vi "gjson_Flatten.vi"(5 "Encap'd by Array?":bool=TRUE, 7 "FlattenedData":string, 8 "error in":errorcluster, 9 "offset (0)":i32, 10 "Variant":variant, 11 "JSON String In":string) -> (0 "error out":errorcluster, 1 "offset out":i32, 3 "JSON String Out":string)   [LabVIEW 2015, in "Json2Labv.lvlib"]
doc: "This recursive VI is the core engine responsible for converting the LabVIEW cluster into an JSON string. \n\nThe VI identifies the top level datatype of the input variant and recursively calls itself when an encapsulaing datatype is found (ie cluster or array). When a fundamental item is found (integer, boolean, etc) it is converted to text and given tags with appropriate attributes and hierarchy."
uses:
  Json2Labv.lvlib
  <vilib>/Utility/VariantDataType/VariantType.lvlib
  <vilib>/Utility/Data Type/NI_Data Type.lvlib
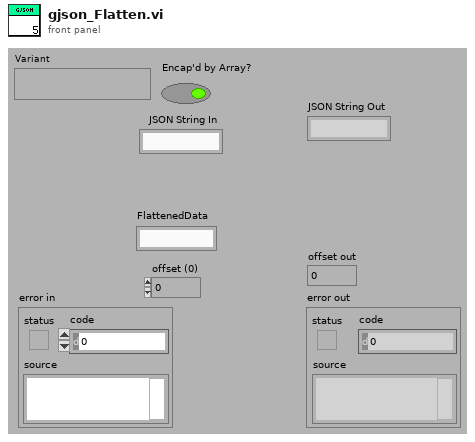
[diagram p1: front panel]
types:
  T1 = typedef "NI_Data Type.lvlib/Data Type.ctl" = enum8{"Invalid Type", "Void", "I8", "I16", "I32", "I64", "U8", "U16", "U32", "U64", "Single Float", "Double Float", "Extended Float", "Single Complex", "Double Complex", "Extended Complex", "Enum U8", "Enum U16", "Enum U32", "Enum U64", "Single Float With Unit", "Double Float With Unit", "Extended Float With Unit", "Single Complex with Unit", "Double Complex with Unit", "Extended Complex with Unit", "Boolean", "String", "Path", "Picture", "Tag", "Array", "Cluster", "Variant", "LV Variant", "Waveform", "Timestamp", "Digital Waveform", "Digital Data", "ExpressData", "Refnum", "External Data", "VI", "Poly VI", "LabVIEW Class Instance", "Fixed Point"}
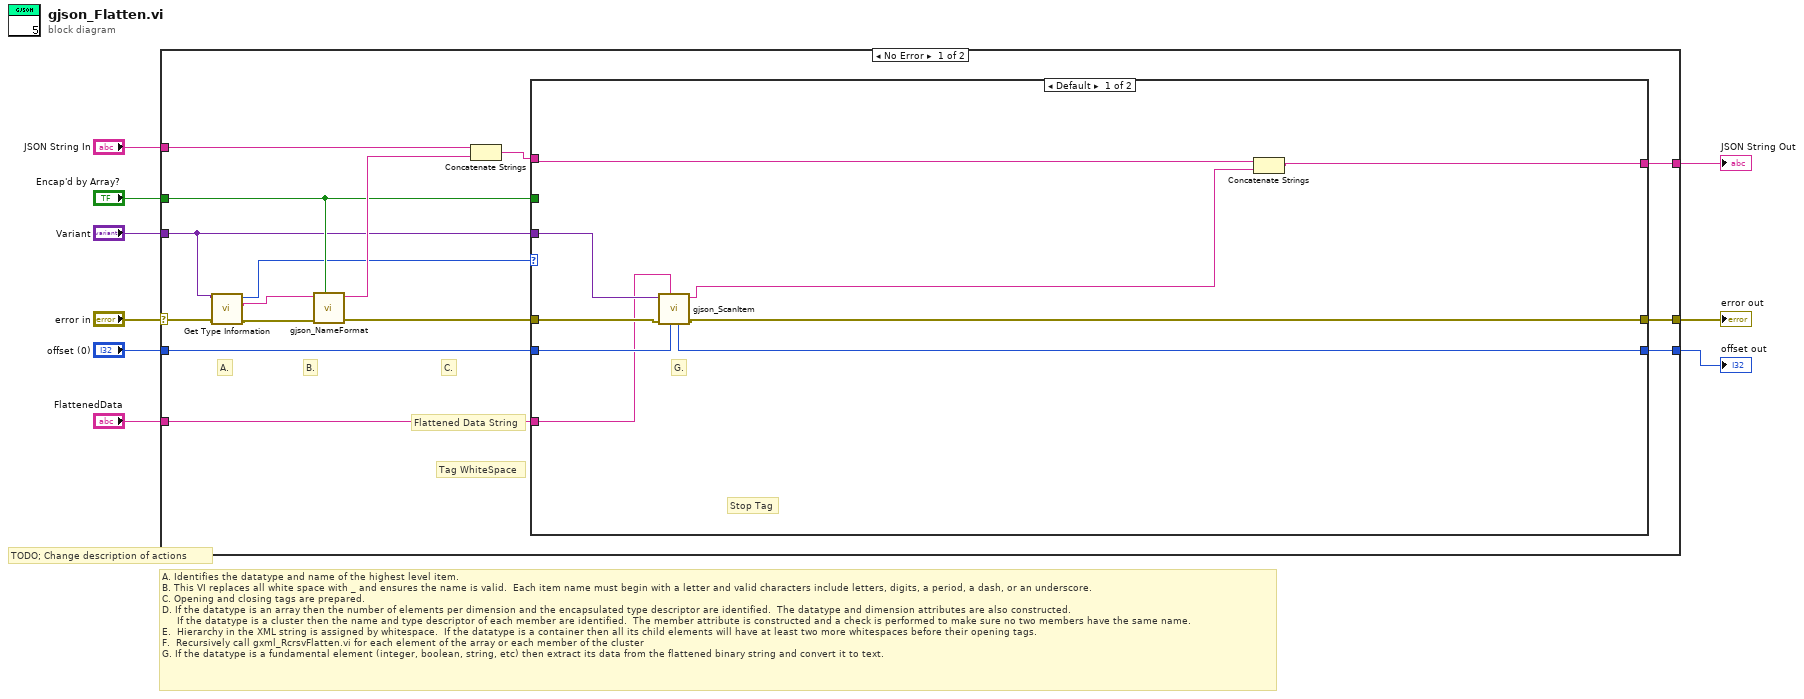
[diagram p0: block diagram]
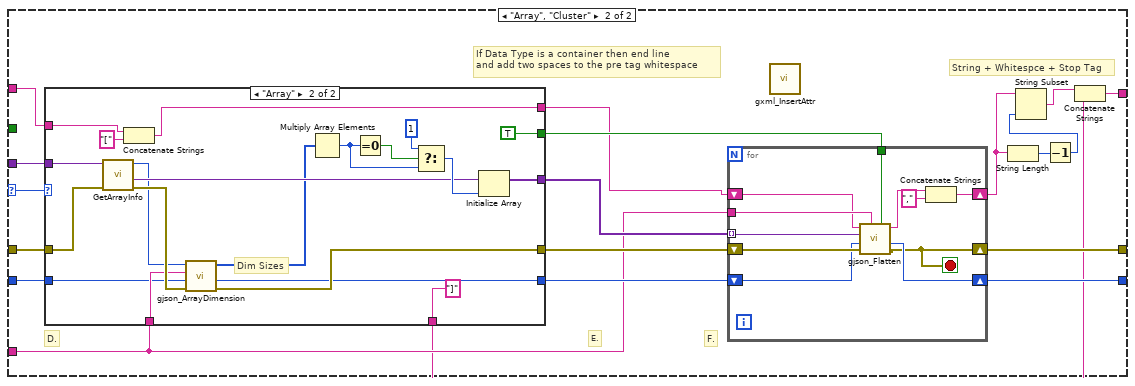
[diagram p2: hidden frame]
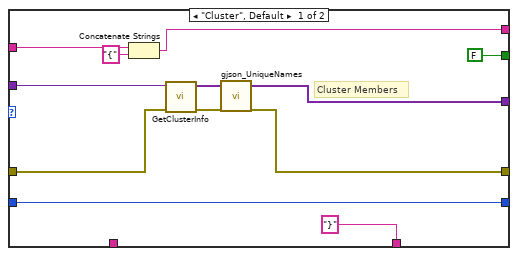
[diagram p3: hidden frame]
diagram:
  # "TODO; Change description of actions"
  # "A. Identifies the datatype and name of the highest level item.\nB. This VI replaces all white space with _ and ensures the name is valid.  Each item name must begin with a letter and valid characters include letters, digits, a period, a dash, or an underscore.\nC. Opening and closing tags are prepared.\nD. If the datatype is an array then the number of elements per dimension and the encapsulated type descriptor are identified.  The datatype and dimension attributes are also constructed.\n     If the datatype is a cluster then the name and type descriptor of each member are identified.  The member attribute is constructed and a check is performed to make sure no two members have the same name.\nE.  Hierarchy in the XML string is assigned by whitespace.  If the datatype is a container then all its child elements will have at least two more whitespaces before their opening tags.\nF.  Recursively call gxml_RcrsvFlatten.vi for each element of the array or each member of the cluster\nG. If the datatype is a fundamental element (integer, boolean, string, etc) then extract its data from the flattened binary string and convert it to text."
  n1 = case shown="No Error" "error in" {
    selector: "error in" -> [w13 w98]
    tunnel: [w24 w98] -> w9
    tunnel: [w22 w97] -> w6
    tunnel: [w23 w96] -> w3
    tunnel: "JSON String In" -> [w17 w97]
    tunnel: "Encap'd by Array?" -> [w15 _]
    tunnel: "offset (0)" -> [w20 w96]
    tunnel: "Variant" -> [w14 _]
    tunnel: "FlattenedData" -> [w19 _]
    frame No Error {
      # "C."
      # "B."
      # "A."
      # "Flattened Data String"
      # "Tag WhiteSpace"
      n2 = call <vilib>:"Get Type Information.vi"("error in (no error)"=w13, "Variant"=w14) -> ("error out"=w10:errorcluster, "Name"=w11:string, "Type"=w12:T1)  [unwired: 5 in, 2 out]
      n3 = call "gjson_NameFormat.vi"("Encap'd by Array?"=w15, "error in"=w10, "JSON String"=w11) -> ("error out"=w18:errorcluster, "JSON_String"=w16:string)  [unwired: 7 in]
      n4 = Concatenate Strings(w17, w16) -> (w21:string)
      n5 = case shown="Default" w12 {
        selector: w12 -> [_ w47]
        tunnel: w14 -> [w29 w52]
        tunnel: w18 -> [w32 w51]
        tunnel: [w27 w40] -> w22
        tunnel: w20 -> [w31 w50]
        tunnel: [w33 w46] -> w24
        tunnel: [w30 w45] -> w23
        tunnel: w21 -> [w25 w42]
        tunnel: w15 -> [_ _]
        tunnel: w19 -> [w28 w39]
        frame Default {
          # "G."
          # "Stop Tag"
          n6 = call "gjson_ScanItem.vi"("Offset In"=w31, "FlattenedData"=w28, "error in"=w32, "variant"=w29) -> ("error out"=w33:errorcluster, "DataString"=w26:string, "Offset Out"=w30:i32)  [unwired: 4 in, 1 out]
          n7 = Concatenate Strings(w25, w26) -> (w27:string)
        }
        frame "Array", "Cluster" {
          # "E."
          # "F."
          # "D."
          # "If Data Type is a container then end line\nand add two spaces to the pre tag whitespace"
          # "String + Whitespce + Stop Tag"
          n8 = case shown="\"Array\"" w47 {
            tunnel: w52 -> [w61 w77]
            tunnel: w51 -> [w62 w78]
            tunnel: w50 -> [w63 w65]
            tunnel: [w58 w84] -> w49
            tunnel: [w57 w71] -> w48
            tunnel: [FALSE TRUE] -> w44
            tunnel: [w63 w70] -> w43
            tunnel: w39 -> [_ w66]
            tunnel: w42 -> [w56 w74]
            tunnel: [w54 w73] -> w41
            tunnel: ["}" ("string") "]" ("string")] -> w34
            frame "Cluster", Default {
              # "Cluster Members"
              n9 = Concatenate Strings(w56, "{" ("string")) -> (w54:string)
              n10 = call <vilib>:"GetClusterInfo.vi"("error in (no error)"=w62, "Variant"=w61) -> ("error out"=w59:errorcluster, "Cluster Elements"=w60:variant[])  [unwired: 8 in]
              n11 = call "gjson_UniqueNames.vi"("error in"=w59, "Cluster Elements"=w60) -> ("error out"=w57:errorcluster, "Cluster Elements Out"=w58:variant[])  [unwired: 8 in]
            }
            frame "Array" {
              # "Dim Sizes"
              n12 = call <vilib>:"GetArrayInfo.vi"("error in (no error)"=w78, "Variant"=w77) -> ("error out"=w68:errorcluster, "ArrayElement"=w76:variant, "NDims"=w67:i32)  [unwired: 6 in, 1 out]
              n13 = Concatenate Strings(w74, "[" ("string")) -> (w73:string)
              n14 = call "gjson_ArrayDimension.vi"("error in"=w68, "offset (0)"=w65, "Flattened Data String"=w66, "Dimensions"=w67) -> ("error out"=w71:errorcluster, "offset"=w70:i32, "ArrayDimensions"=w69:i32[])  [unwired: 4 in, 1 out]
              n15 = Multiply Array Elements(1:w69) -> (0:w82:i32)
              n16 = Equal To 0?(x=w82) -> (x = 0?=w83:bool)
              n17 = Select(t=1, s=w83, f=w82) -> (s? t:f=w80:i32)
              n18 = Initialize Array(w76, w80) -> (w84:variant[])
            }
          }
          n19 = for {
            shift-right: [w86] -> w38
            shift-left: w41 -> [w89]
            shift-right: [w95] -> w45
            shift-left: w43 -> [w92]
            tunnel: w49 -> [w88] mode=indexing
            tunnel: w44 -> [w91]
            shift-right: [w94] -> w46
            shift-left: w48 -> [w93]
            tunnel: w39 -> [w90]
            stop <- w94 stop-if-true
            n20 = call "gjson_Flatten.vi"("Encap'd by Array?"=w91, "FlattenedData"=w90, "error in"=w93, "offset (0)"=w92, "Variant"=w88, "JSON String In"=w89) -> ("error out"=w94:errorcluster, "offset out"=w95:i32, "JSON String Out"=w87:string)  [unwired: 3 in]
            n21 = Concatenate Strings(w87, "," ("string")) -> (w86:string)
          }
          n22 = call "gxml_InsertAttr.vi"() -> ()  [unwired: 5 in, 1 out]
          n23 = String Length(string=w38) -> (length=w37:i32)
          n24 = Decrement(x=w37) -> (x-1=w36:i32)
          n25 = String Subset(string=w38, length (rest)=w36) -> (substring=w35:string)  [unwired: 1 in]
          n26 = Concatenate Strings(w35, w34) -> (w40:string)
        }
      }
    }
    frame Error {
    }
  }
  "error out" <- w9
  "JSON String Out" <- w6
  "offset out" <- w3
